vi "Send xps_panel_generate_pvt_trajectory.vi"(5 "custom?":bool, 7 "Message Priority (Normal)":T3=enum."Normal", 8 "error in (no error)":errorcluster, 9 "Dither Cycles":u32=3, 10 "Custom Dither Trajectory":T1 {"Dither Period (s)" min=0.0; "PVT Ampl (nm)" min=0.0}, 11 "Message Enqueuer":refnum<class "Message Enqueuer.lvclass">) -> (0 "error out":errorcluster, 3 "Message Enqueuer out":refnum<class "Message Enqueuer.lvclass">)   [LabVIEW 2015, in "xps_panel_generate_pvt_trajectory Msg.lvclass"]
doc: "This VI sends the message to an actor."
uses:
  xps_panel_generate_pvt_trajectory Msg.lvclass
  <vilib>/ActorFramework/Message Enqueuer/Message Enqueuer.lvclass
  <vilib>/ActorFramework/Message Enqueuer/Message Priority.ctl
  newport_xps/dither_trajectory_settings.ctl
  newport_xps/dither_trajectory_types.ctl
  xps_panel_generate_pvt_trajectory Msg.lvclass/xps_panel_generate_pvt_trajectory Msg.ctl
  <vilib>/ActorFramework/Message Enqueuer/Message Enqueuer.lvclass/Message Enqueuer.ctl
  <vilib>/ActorFramework/Message Priority Queue/Priority Enqueue.vi
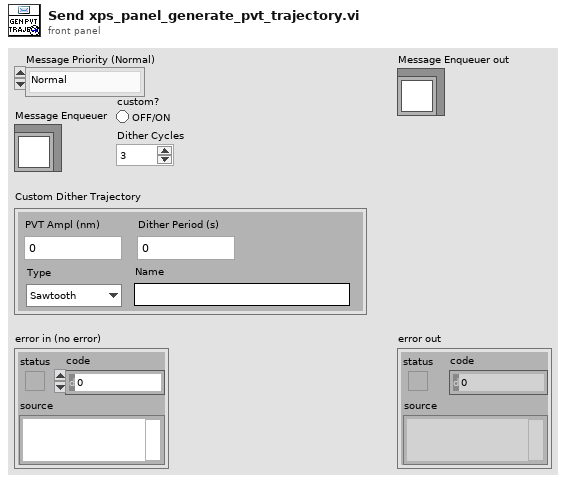
[diagram p1: front panel]
types:
  T1 = typedef "dither_trajectory_settings.ctl" = cluster{"PVT Ampl (nm)":dbl, "Dither Period (s)":dbl, "Type":T2, "Name":string}
  T2 = typedef "dither_trajectory_types.ctl" = enum16{"Sawtooth"}
  T3 = typedef "Actor Framework.lvlib/Message Enqueuer.lvclass/Message Priority.ctl" = enum16{"Low", "Normal", "High"}
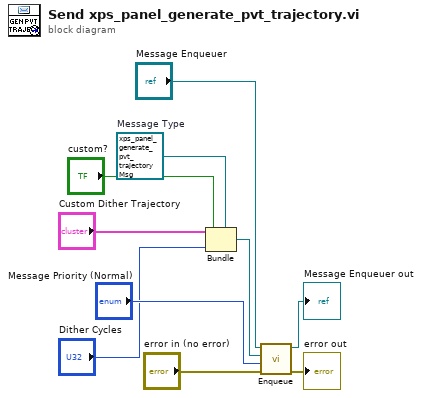
[diagram p0: block diagram]
diagram:
  w7 = refnum<class "xps_panel_generate_pvt_trajectory Msg.lvclass"> refnum  # Message Type
  n1 = Bundle(cluster=w7, "Custom Dither Trajectory", "custom?", "Dither Cycles") -> (w6:refnum<class "xps_panel_generate_pvt_trajectory Msg.lvclass">)
  n2 = call <vilib>:"Enqueue.vi"("error in (no error)"="error in (no error)", "Message Priority (Normal)"="Message Priority (Normal)", "Message"=w6, "Message Enqueuer in"="Message Enqueuer") -> ("error out"=→"error out":errorcluster, "Message Enqueuer out"=→"Message Enqueuer out":refnum<class "Message Enqueuer.lvclass">)  [unwired: 6 in]
